vi "Lift Execute.vi"() -> ()   [LabVIEW 2017]
uses:
  Lift Control Type.ctl
  Brake Enum States.ctl
  <vilib>/Rock Robotics/WPI/DriverStation/WPI_DriverStationRobotMode2.ctl
  <vilib>/Rock Robotics/WPI/Solenoid/WPI_SolenoidValue.ctl
  Lift Notifier.ctl
  Lift Enum States.ctl
  <vilib>/Rock Robotics/WPI/ThirdParty/Phoenix-LabVIEW/Motor Controller/Controls/CTRE_Phoenix_MotorControl_ControlMode.ctl
  Lift Globals.vi
  Utility VIs/Refnum Names.vi
  Robot Global Data.vi
  <vilib>/Rock Robotics/WPI/ThirdParty/Phoenix-LabVIEW/Motor Controller/Get/CTRE_Phoenix_MotorController_GetOutputCurrent_Enhanced.vi
  <vilib>/Rock Robotics/Network Tables/NT Write Number.vi
  <vilib>/Rock Robotics/Network Tables/NT Write Boolean.vi
  <vilib>/Rock Robotics/WPI/Solenoid/WPI_SolenoidSetEnum.vi
panel:
  in  "Switch Add":dbl=1000.0 format="%#_13g"
  in  "Portal":dbl=4750.0
  out "Counts Met":bool=TRUE
  in  "Counts":i32=15
  out "Output":dbl(graph)
  in  "Graphs":bool=TRUE
  out "Position":i32(graph)
  out "Current":T1(graph)
  in  "Lift Allowable Error Down":dbl=100.0
  out "Current Error":dbl
  in  "kP Max Down":dbl=-1.0
  in  "kP Max Up":dbl=1.0
  in  "Lift Allowable Error Up":dbl=100.0
  in  "kP Down":dbl=4.18e-05
  in  "kP Up":dbl=0.00017
  out "error out 5":errorcluster
  out "error out 4":errorcluster={"status"=TRUE, "code"=-44047, "source"="Solenoid 5<LOCATION>Lift Execute.vi<CALLSTACK>Lift Execute.vi< <Periodic Tasks.vi< <Robot Main.vi"}
  out "error out 3":errorcluster={"status"=TRUE, "code"=1, "source"="Wait on Notification in Lift Execute.vi->Periodic Tasks.vi->Robot Main.vi"}
  out "error out 2":errorcluster
  out "error out":errorcluster={"status"=TRUE, "code"=1, "source"="Wait on Notification in Lift Execute.vi->Periodic Tasks.vi->Robot Main.vi"}
  in  "Deadband 2":i32=6000
  in  "Deadband 1":i32=300
  in  "Drive Up Time (ms)":u32=100
  in  "Brake Disengage Time":u32=100
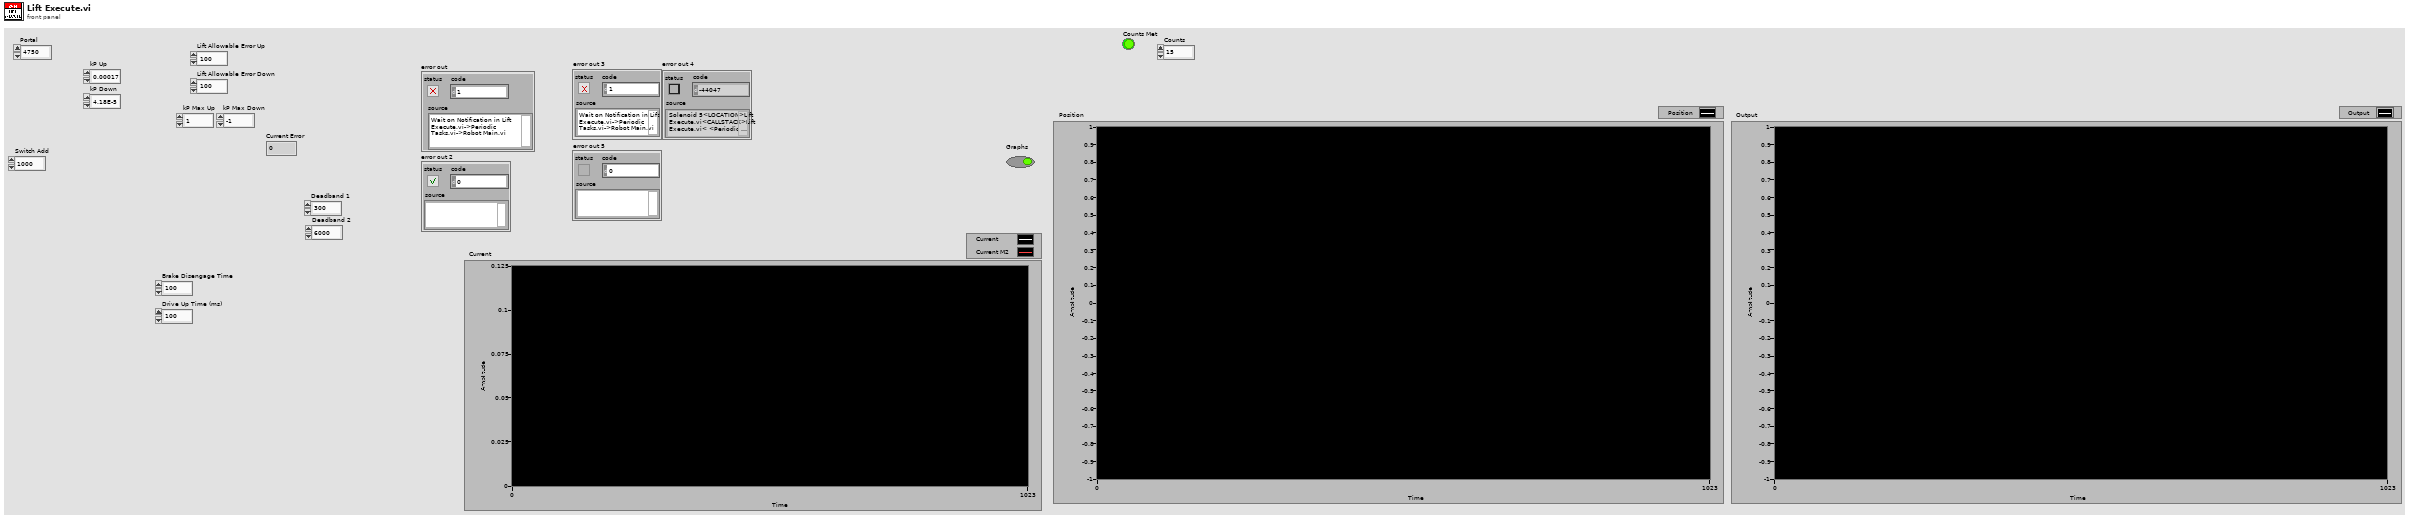
[diagram p1: front panel]
types:
  T1 = cluster{"Output Current":dbl, "Output Current":dbl}
  T2 = typedef "WPI_MotorControlDeviceRef.ctl" = cluster{"DeviceStatus":errorcluster, "Type":T3, "PWM":cluster{"PWM Channel":T4, "DeadBand":T5}, "CAN":cluster{"Device Number":u8, "SetOutput VI Ref":variant, "GetOutput VI Ref":variant, "Enable VI Ref":variant, "Disable VI Ref":variant, "Data":variant}, "Invert":bool, "DIO PWM":cluster{"PWM \"Enable\" Channel":T4, "DIOChannel":T6, "PWM Rate":dbl}}
  T3 = typedef "WPI_MotorControlType.ctl" = enum16{"PWM", "CAN", "DIO PWM"}
  T4 = typedef "FPGA_DIOPWMChannel.ctl" = enum8{"PWM 0", "PWM 1", "PWM 2", "PWM 3", "PWM 4", "PWM 5", "PWM 6", "PWM 7", "PWM 8", "PWM 9", "PWM MXP 0", "PWM MXP 1", "PWM MXP 2", "PWM MXP 3", "PWM MXP 4", "PWM MXP 5", "PWM MXP 6", "PWM MXP 7", "PWM MXP 8", "PWM MXP 9", "Invalid"}
  T5 = typedef "WPI_PWMDeadband.ctl" = cluster{"Name":string, "maxPositivePwm":i32, "minPositivePwm":i32, "centerPwm":i32, "maxNegativePwm":i32, "minNegativePwm":i32, "angularRange":u16}
  T6 = typedef "FPGA_DIOChannel.ctl" = enum8{"DIO 0", "DIO 1", "DIO 2", "DIO 3", "DIO 4", "DIO 5", "DIO 6", "DIO 7", "DIO 8", "DIO 9", "DIO MXP 0", "DIO MXP 1", "DIO MXP 2", "DIO MXP 3", "DIO MXP 4", "DIO MXP 5", "DIO MXP 6", "DIO MXP 7", "DIO MXP 8", "DIO MXP 9", "DIO MXP 10", "DIO MXP 11", "DIO MXP 12", "DIO MXP 13", "DIO MXP 14", "DIO MXP 15", "SPI Port CS1", "SPI Port CS2", "SPI Port CS3", "SPI Port MISO", "SPI Port MOSI", "Invalid"}
  T7 = typedef "WPI_SolenoidDevRef.ctl" = cluster{"DevStatus":errorcluster, "Pneumatics Control Module":u8, "Forward Solenoid Channel":T8, "Reverse Solenoid Channel":T8}
  T8 = typedef "WPI_SolenoidChannel.ctl" = enum8{"Solenoid 0", "Solenoid 1", "Solenoid 2", "Solenoid 3", "Solenoid 4", "Solenoid 5", "Solenoid 6", "Solenoid 7", "Invalid"}
  T9 = typedef "WPI_SolenoidValue.ctl" = enum16{"Off", "On", "Forward", "Reverse"}
  T10 = typedef "Lift Control Type.ctl" = enum16{"No Op", "Position", "Climb Actuation", "Manual Up", "Manual Down", "PositionAuto", "Position_kP", "Position_Delay"}
  T11 = typedef "WPI_DriverStationRobotMode2.ctl" = enum16{"Autonomous Disabled", "Autonomous Enabled", "Teleop Disabled", "Teleop Enabled", "Disconnected", "Finish", "Test Disabled", "Test Enabled", "Emergency Stopped"}
  T12 = typedef "Brake Enum States.ctl" = enum16{"Brake", "Disengage Brake", "Drive Up", "Pass Through"}
  T13 = typedef "Lift Notifier.ctl" = cluster{"Lift Control Type":T10, "Step":i32, "Set Position":T14, "Climb":bool, "Switch":bool, "Scale Low":bool, "Scale Mid":bool, "Scale High":bool, "Stow":bool, "Load":bool, "Climb Actuation":bool, "Manual Up":bool, "Manual Down":bool, "Parameter 1":dbl, "Parameter 2":dbl, "Parameter 3":dbl, "Lift Notifier":refnum<notifier>, "Exchange":bool, "Brake":bool, "Portal":bool}
  T14 = typedef "Lift Enum States.ctl" = enum16{"Climb", "Load", "Portal", "Switch", "Scale High", "Scale Mid", "Scale Low", "Exchange", "Stow", "Current Position"}
  T15 = typedef "CTRE_Phoenix_MotorControl_ControlMode.ctl" = u16
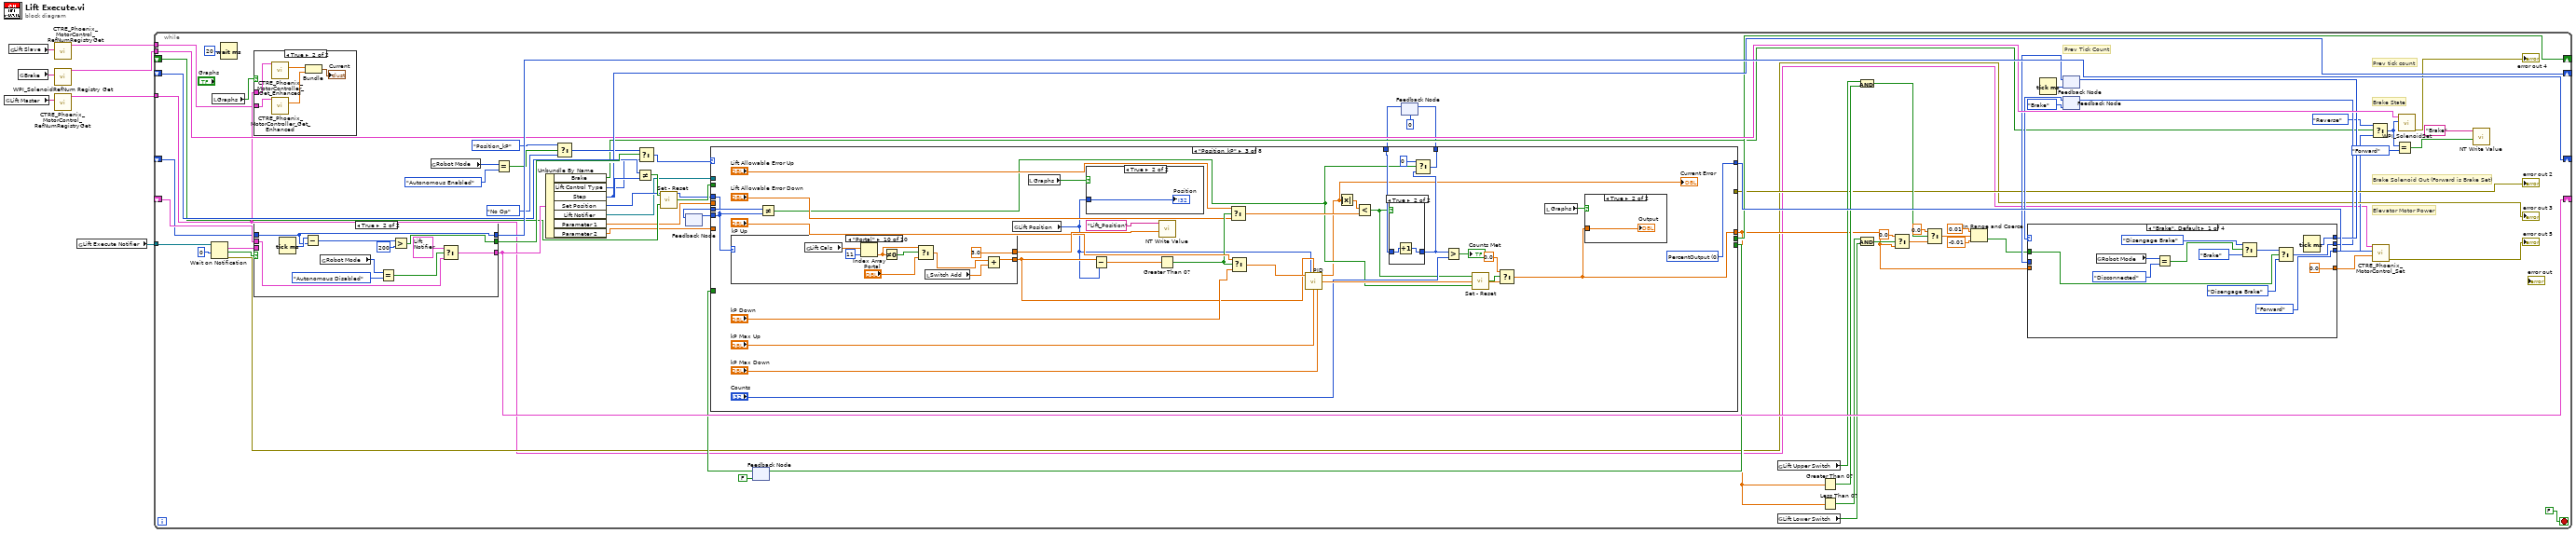
[diagram p0: block diagram]
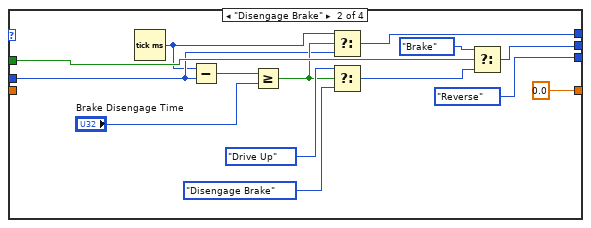
[diagram p3: hidden frame]
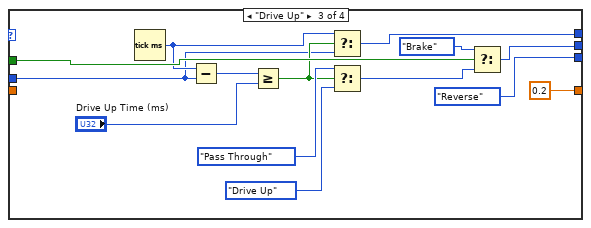
[diagram p4: hidden frame]
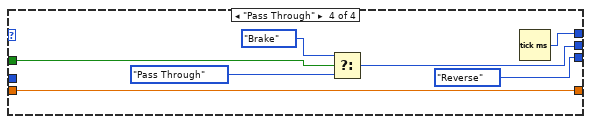
[diagram p5: hidden frame]
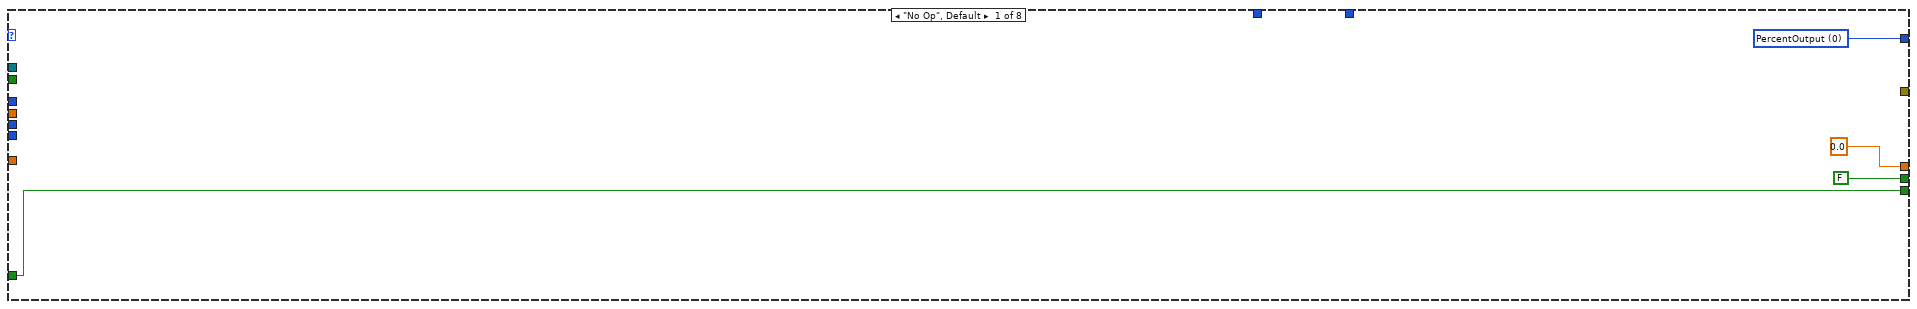
[diagram p6: hidden frame]
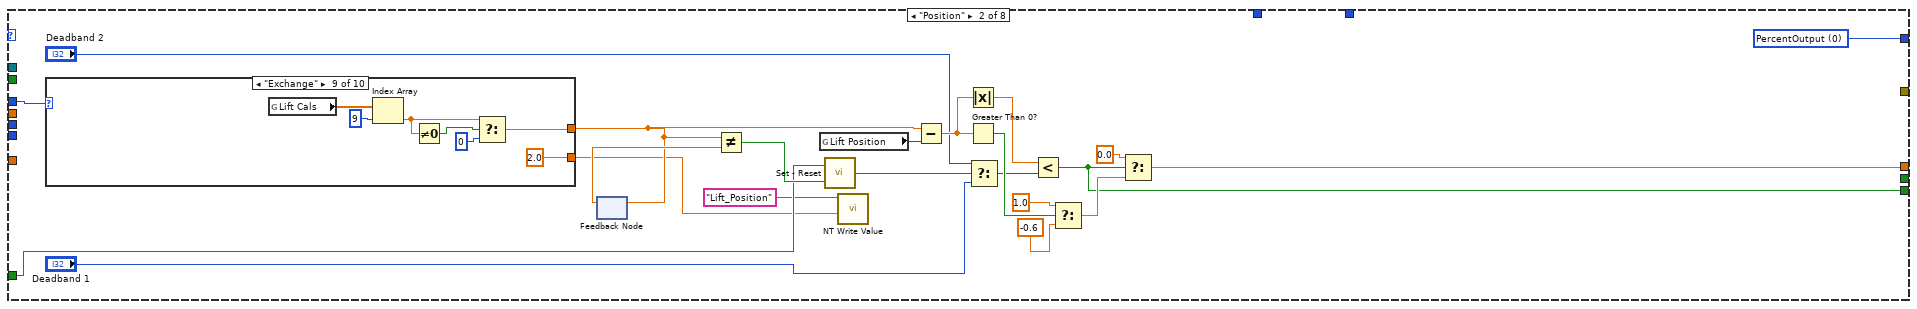
[diagram p7: hidden frame]
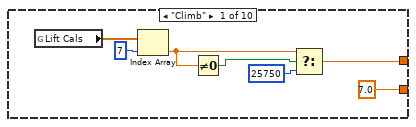
[diagram p8: hidden frame]
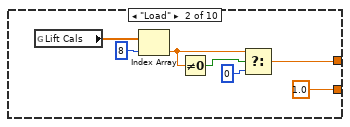
[diagram p9: hidden frame]
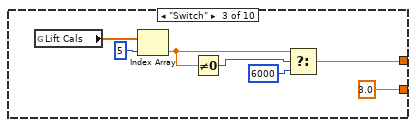
[diagram p10: hidden frame]
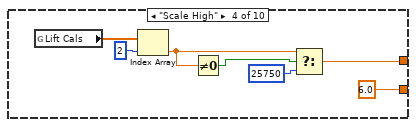
[diagram p11: hidden frame]
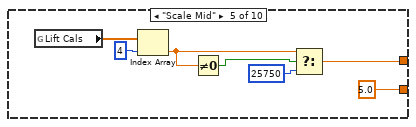
[diagram p12: hidden frame]
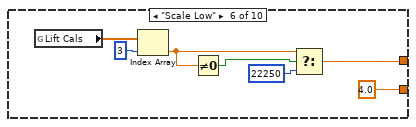
[diagram p13: hidden frame]
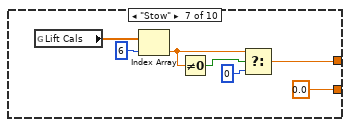
[diagram p14: hidden frame]
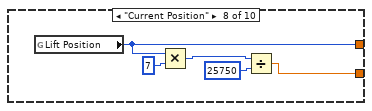
[diagram p15: hidden frame]
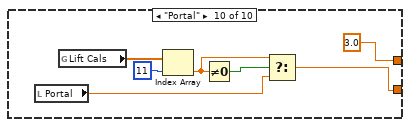
[diagram p16: hidden frame]
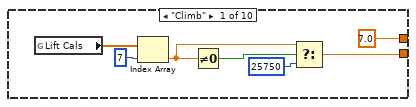
[diagram p20: hidden frame]
diagram:
  n1 = global read "Refnum Names.vi" "Lift Master"() -> (w6:string)
  n2 = global read "Refnum Names.vi" "Lift Slave"() -> (w2:string)
  n3 = global read "Refnum Names.vi" "Brake"() -> (w4:string)
  n4 = call <vilib>:"CTRE_Phoenix_MotorControl_RefNumRegistryGet.vi"("refnum name"=w2) -> ("PhoenixMotorControlDevRef"=w1:T2)  [unwired: 9 in, 1 out]
  n5 = call <vilib>:"WPI_SolenoidRefNum Registry Get.vi"("refnum name"=w4) -> ("SolenoidDevRef"=w3:T7)  [unwired: 9 in, 1 out]
  n6 = call <vilib>:"CTRE_Phoenix_MotorControl_RefNumRegistryGet.vi"("refnum name"=w6) -> ("PhoenixMotorControlDevRef"=w5:T2)  [unwired: 9 in, 1 out]
  n7 = global read "Lift Globals.vi" "Lift Execute Notifier"() -> (w7:refnum<notifier>)
  n8 = while {
    tunnel: w7 -> [w79]
    shift-right: [w68] -> _
    shift-left: _ -> [w76]
    shift-right: [w74] -> _
    shift-left: _ -> [w64]
    shift-right: [w71] -> _
    shift-left: _ -> [w72]
    tunnel: w5 -> [w15]
    tunnel: w3 -> [w65]
    shift-right: [w63] -> _
    shift-left: _ -> [w62]
    tunnel: w1 -> [w14]
    stop <- FALSE stop-if-true
    # "Elevator Motor Power"
    # "Prev tick count"
    # "Brake State"
    # "Brake Solenoid Out (Forward is Brake Set)"
    # "Prev Tick Count"
    n9 = Wait on Notification(notifier=w79, timeout in ms (-1)=0) -> (notification=w75:T13, timed out?=w77:bool, error out=→"error out 3":errorcluster)  [unwired: 2 in, 1 out]
    n10 = local read "Graphs"() -> (w13:bool)
    n11 = Wait (ms)(milliseconds to wait=u32 20) -> ()  [unwired: 1 out]
    n12 = case shown="True" w13 {
      tunnel: w15 -> [_ w86]
      tunnel: w14 -> [_ w85]
      frame False {
      }
      frame True {
        n13 = call-poly <vilib>:"CTRE_Phoenix_MotorController_Get_Enhanced.vi"("PhoenixMotorControlDevRef"=w86) -> ("Output Current"=w83:dbl)  [unwired: 12 in, 2 out]
        n14 = call-poly <vilib>:"CTRE_Phoenix_MotorController_Get_Enhanced.vi"("PhoenixMotorControlDevRef"=w85) -> ("Output Current"=w84:dbl)  [unwired: 12 in, 2 out]
        n15 = Bundle("Output Current"=w83, "Output Current"=w84) -> (→"Current":T1)  [unwired: 1 in]
      }
    }
    n16 = case shown="True" w77 {
      tunnel: w76 -> [_ w401]
      tunnel: [w391 w400] -> w68
      tunnel: w75 -> [w391 _]
      tunnel: [w390 w393] -> w74
      tunnel: w64 -> [_ w393]
      tunnel: [FALSE w396] -> w73
      frame False {
        n17 = Tick Count (ms)() -> (millisecond timer value=w390:u32)
      }
      frame True {
        n18 = Tick Count (ms)() -> (millisecond timer value=w399:u32)
        n19 = Subtract(x=w399, y=w393) -> (x-y=w398:u32)
        n20 = global read "Robot Global Data.vi" "Robot Mode"() -> (w395:T11)
        n21 = Equal?(x=w395, y=WPI_DriverStationRobotMode2."Autonomous Disabled") -> (x = y?=w402:bool)
        n22 = Greater?(x=w398, y=u32 200) -> (0:w396:bool)
        n23 = Select(t=T13 {"Lift Control Type"=enum."No Op", "Step"=0, "Set Position"=enum."Load", "Climb"=FALSE, "Switch"=FALSE, "Scale Low"=FALSE, "Scale Mid"=FALSE, "Scale High"=FALSE, "Stow"=FALSE, "Load"=FALSE, "Climb Actuation"=FALSE, "Manual Up"=FALSE, "Manual Down"=FALSE, "Parameter 1"=0.0, "Parameter 2"=0.0, "Parameter 3"=0.0, "Lift Notifier"=refnum, "Exchange"=FALSE, "Brake"=FALSE, "Portal"=FALSE} ("Lift Notifier"), s=w402, f=w401) -> (s? t:f=w400:T13)
      }
    }
    n24 = global read "Robot Global Data.vi" "Robot Mode"() -> (w33:T11)
    n25 = Equal?(x=w33, y=WPI_DriverStationRobotMode2."Autonomous Enabled") -> (x = y?=w34:bool)
    n26 = Unbundle By Name(w68) -> ("Brake"=w20:bool, "Lift Control Type"=w61:T10, "Step"=w71:i32, "Set Position"=w67:T14, "Lift Notifier"=w36:refnum<notifier>, "Parameter 1"=w28:dbl, "Parameter 2"=w16:dbl)
    n27 = Select(t=Lift_Control_Type."Position_kP", s=w34, f=Lift_Control_Type."No Op" ("t")) -> (s? t:f=w29:T10)
    n28 = Not Equal?(x=w72, y=w71) -> (x != y?=w70:bool)
    n29 = Select(t=w29, s=w73, f=w61) -> (s? t:f=w31:T10)
    n30 = call "Set - Reset.vi"("Reset"=w62, "Set"=w70) -> ("Output"=w69:bool)
    n31 = feedback #1() -> (w8:T14)  [unwired: 1 in]
    n32 = feedback #2(FALSE) -> (w49:bool)
    n33 = feedback #3(0) -> (w10:i32)
    n34 = case shown="\"Position_kP\"" w31 {
      tunnel: w69 -> [_ _ _ _ _ _ w376 w382]
      tunnel: w67 -> [_ w143 w237 _ _ _ w377 w381]
      tunnel: [0.0 ("Output") w156 w242 w338 w349 w360 w375 w385] -> w37
      tunnel: [w137 w159 w260 w344 w356 w369 w378 w388] -> w66
      tunnel: [FALSE ("notification") _ _ _ _ FALSE w374 w384] -> w63
      tunnel: [w135 w149 _ _ _ _ _ _] -> w50
      tunnel: w49 -> [w135 w145 _ _ _ _ _ _]
      tunnel: w36 -> [_ _ _ _ _ _ w372 w387]
      tunnel: w28 -> [_ _ _ _ _ _ w371 w380]
      tunnel: [_ _ _ _ _ _ w370 w386] -> w27
      tunnel: w16 -> [_ _ _ _ _ _ _ w379]
      tunnel: [_ _ w235 _ _ _ _ _] -> w11
      tunnel: w10 -> [_ _ w240 _ _ _ _ _]
      tunnel: [_ _ w237 _ _ _ _ _] -> w9
      tunnel: w8 -> [_ _ w238 _ _ _ _ _]
      frame "No Op", Default {
        w137 = T15 0 items=["PercentOutput"=0, "Position"=1, "Velocity"=2, "Current"=3, "Follower"=5, "MotionProfile"=6, "MotionMagic"=7, "MotionMagicArc"=8, "MotionProfileArc"=10, "Disabled"=15] ("Control Mode")
      }
      frame "Position" {
        w159 = T15 0 items=["PercentOutput"=0, "Position"=1, "Velocity"=2, "Current"=3, "Follower"=5, "MotionProfile"=6, "MotionMagic"=7, "MotionMagicArc"=8, "MotionProfileArc"=10, "Disabled"=15] ("Control Mode")
        n35 = case shown="\"Exchange\"" w143 {
          tunnel: [w161 w169 w175 w182 w189 w196 w205 w213 w215 3.0 ("Numeric")] -> w144
          tunnel: [7.0 1.0 3.0 6.0 5.0 4.0 0.0 w209 2.0 w223] -> w139
          frame "Climb" {
            n36 = global read "Lift Globals.vi" "Lift Cals"() -> (w166:dbl[])
            n37 = Index Array(array=w166, index=7) -> (element=w163:dbl)
            n38 = Not Equal To 0?(x=w163) -> (x != 0?=w164:bool)
            n39 = Select(t=w163, s=w164, f=25750 ("Lift Position")) -> (s? t:f=w161:dbl)
          }
          frame "Load" {
            n40 = global read "Lift Globals.vi" "Lift Cals"() -> (w173:dbl[])
            n41 = Index Array(array=w173, index=8) -> (element=w170:dbl)
            n42 = Not Equal To 0?(x=w170) -> (x != 0?=w171:bool)
            n43 = Select(t=w170, s=w171, f=0 ("Lift Position")) -> (s? t:f=w169:dbl)
          }
          frame "Switch" {
            n44 = global read "Lift Globals.vi" "Lift Cals"() -> (w180:dbl[])
            n45 = Index Array(array=w180, index=5) -> (element=w176:dbl)
            n46 = Not Equal To 0?(x=w176) -> (x != 0?=w178:bool)
            n47 = Select(t=w176, s=w178, f=6000 ("Lift Position")) -> (s? t:f=w175:dbl)
          }
          frame "Scale High" {
            n48 = global read "Lift Globals.vi" "Lift Cals"() -> (w187:dbl[])
            n49 = Index Array(array=w187, index=2) -> (element=w183:dbl)
            n50 = Not Equal To 0?(x=w183) -> (x != 0?=w185:bool)
            n51 = Select(t=w183, s=w185, f=25750 ("Lift Position")) -> (s? t:f=w182:dbl)
          }
          frame "Scale Mid" {
            n52 = global read "Lift Globals.vi" "Lift Cals"() -> (w194:dbl[])
            n53 = Index Array(array=w194, index=4) -> (element=w190:dbl)
            n54 = Not Equal To 0?(x=w190) -> (x != 0?=w192:bool)
            n55 = Select(t=w190, s=w192, f=25750 ("Lift Position")) -> (s? t:f=w189:dbl)
          }
          frame "Scale Low" {
            n56 = global read "Lift Globals.vi" "Lift Cals"() -> (w201:dbl[])
            n57 = Index Array(array=w201, index=3) -> (element=w197:dbl)
            n58 = Not Equal To 0?(x=w197) -> (x != 0?=w199:bool)
            n59 = Select(t=w197, s=w199, f=22250 ("Lift Position")) -> (s? t:f=w196:dbl)
          }
          frame "Stow" {
            n60 = global read "Lift Globals.vi" "Lift Cals"() -> (w208:dbl[])
            n61 = Index Array(array=w208, index=6) -> (element=w204:dbl)
            n62 = Not Equal To 0?(x=w204) -> (x != 0?=w206:bool)
            n63 = Select(t=w204, s=w206, f=0 ("Lift Position")) -> (s? t:f=w205:dbl)
          }
          frame "Current Position" {
            n64 = global read "Lift Globals.vi" "Lift Position"() -> (w213:i32)
            n65 = Multiply(x=w213, y=7) -> (x*y=w211:i32)
            n66 = Divide(x=w211, y=25750) -> (x/y=w209:dbl)
          }
          frame "Exchange" {
            n67 = global read "Lift Globals.vi" "Lift Cals"() -> (w220:dbl[])
            n68 = Index Array(array=w220, index=9) -> (element=w216:dbl)
            n69 = Not Equal To 0?(x=w216) -> (x != 0?=w218:bool)
            n70 = Select(t=w216, s=w218, f=0 ("Lift Position")) -> (s? t:f=w215:dbl)
          }
          frame "Portal" {
            n71 = local read "Portal"() -> (w222:dbl)
            n72 = global read "Lift Globals.vi" "Lift Cals"() -> (w227:dbl[])
            n73 = Index Array(array=w227, index=11) -> (element=w224:dbl)
            n74 = Not Equal To 0?(x=w224) -> (x != 0?=w225:bool)
            n75 = Select(t=w224, s=w225, f=w222) -> (s? t:f=w223:dbl)
          }
        }
        n76 = feedback #4() -> (w148:dbl)  [unwired: 1 in]
        n77 = feedback-in #4(w144) -> ()
        n78 = Not Equal?(x=w144, y=w148) -> (x != y?=w146:bool)
        n79 = global read "Lift Globals.vi" "Lift Position"() -> (w158:i32)
        n80 = call "Set - Reset.vi"("Reset"=w146, "Set"=w145) -> ("Output"=w147:bool)
        n81 = call-poly <vilib>:"NT Write Value.vi"("Numeric"=w139, "Name"="Lift_Position") -> ()  [unwired: 9 in, 1 out]
        n82 = Subtract(x=w144, y=w158) -> (x-y=w153:dbl)
        n83 = Absolute Value(x=w153) -> (abs(x)=w150:dbl)
        n84 = Greater Than 0?(x=w153) -> (x > 0?=w157:bool)
        n85 = Select(t="Deadband 2", s=w147, f="Deadband 1") -> (s? t:f=w151:i32)
        n86 = Less?(x=w150, y=w151) -> (x < y?=w149:bool)
        n87 = Select(t=1.0 ("f"), s=w157, f=-0.6) -> (s? t:f=w155:dbl)
        n88 = Select(t=0.0, s=w149, f=w155) -> (s? t:f=w156:dbl)
      }
      frame "Position_kP" {
        w260 = T15 0 items=["PercentOutput"=0, "Position"=1, "Velocity"=2, "Current"=3, "Follower"=5, "MotionProfile"=6, "MotionMagic"=7, "MotionMagicArc"=8, "MotionProfileArc"=10, "Disabled"=15] ("Control Mode")
        n89 = case shown="\"Portal\"" w237 {
          tunnel: [w267 w275 w281 w290 w297 w304 w313 w321 w323 w330] -> w251
          tunnel: [7.0 1.0 3.0 6.0 5.0 4.0 0.0 w317 2.0 3.0] -> w258
          frame "Climb" {
            n90 = global read "Lift Globals.vi" "Lift Cals"() -> (w272:dbl[])
            n91 = Index Array(array=w272, index=7) -> (element=w269:dbl)
            n92 = Not Equal To 0?(x=w269) -> (x != 0?=w270:bool)
            n93 = Select(t=w269, s=w270, f=25750 ("Lift Position")) -> (s? t:f=w267:dbl)
          }
          frame "Load" {
            n94 = global read "Lift Globals.vi" "Lift Cals"() -> (w279:dbl[])
            n95 = Index Array(array=w279, index=8) -> (element=w276:dbl)
            n96 = Not Equal To 0?(x=w276) -> (x != 0?=w277:bool)
            n97 = Select(t=w276, s=w277, f=0 ("Lift Position")) -> (s? t:f=w275:dbl)
          }
          frame "Switch" {
            n98 = global read "Lift Globals.vi" "Lift Cals"() -> (w288:dbl[])
            n99 = Index Array(array=w288, index=5) -> (element=w284:dbl)
            n100 = Not Equal To 0?(x=w284) -> (x != 0?=w286:bool)
            n101 = Select(t=w284, s=w286, f=6000 ("Lift Position")) -> (s? t:f=w283:dbl)
            n102 = Add(x=w283, y="Switch Add") -> (x+y=w281:dbl)
          }
          frame "Scale High" {
            n103 = global read "Lift Globals.vi" "Lift Cals"() -> (w295:dbl[])
            n104 = Index Array(array=w295, index=2) -> (element=w291:dbl)
            n105 = Not Equal To 0?(x=w291) -> (x != 0?=w293:bool)
            n106 = Select(t=w291, s=w293, f=25750 ("Lift Position")) -> (s? t:f=w290:dbl)
          }
          frame "Scale Mid" {
            n107 = global read "Lift Globals.vi" "Lift Cals"() -> (w302:dbl[])
            n108 = Index Array(array=w302, index=4) -> (element=w298:dbl)
            n109 = Not Equal To 0?(x=w298) -> (x != 0?=w300:bool)
            n110 = Select(t=w298, s=w300, f=25750 ("Lift Position")) -> (s? t:f=w297:dbl)
          }
          frame "Scale Low" {
            n111 = global read "Lift Globals.vi" "Lift Cals"() -> (w309:dbl[])
            n112 = Index Array(array=w309, index=3) -> (element=w305:dbl)
            n113 = Not Equal To 0?(x=w305) -> (x != 0?=w307:bool)
            n114 = Select(t=w305, s=w307, f=22250 ("Lift Position")) -> (s? t:f=w304:dbl)
          }
          frame "Stow" {
            n115 = global read "Lift Globals.vi" "Lift Cals"() -> (w316:dbl[])
            n116 = Index Array(array=w316, index=6) -> (element=w312:dbl)
            n117 = Not Equal To 0?(x=w312) -> (x != 0?=w314:bool)
            n118 = Select(t=w312, s=w314, f=0 ("Lift Position")) -> (s? t:f=w313:dbl)
          }
          frame "Current Position" {
            n119 = global read "Lift Globals.vi" "Lift Position"() -> (w321:i32)
            n120 = Multiply(x=w321, y=7) -> (x*y=w319:i32)
            n121 = Divide(x=w319, y=25750) -> (x/y=w317:dbl)
          }
          frame "Exchange" {
            n122 = global read "Lift Globals.vi" "Lift Cals"() -> (w328:dbl[])
            n123 = Index Array(array=w328, index=9) -> (element=w324:dbl)
            n124 = Not Equal To 0?(x=w324) -> (x != 0?=w326:bool)
            n125 = Select(t=w324, s=w326, f=0 ("Lift Position")) -> (s? t:f=w323:dbl)
          }
          frame "Portal" {
            n126 = global read "Lift Globals.vi" "Lift Cals"() -> (w336:dbl[])
            n127 = Index Array(array=w336, index=11) -> (element=w333:dbl)
            n128 = Not Equal To 0?(x=w333) -> (x != 0?=w334:bool)
            n129 = Select(t=w333, s=w334, f="Portal") -> (s? t:f=w331:dbl)
            n130 = local read "Switch Add"() -> (w329:dbl)
            n131 = Add(x=w331, y=w329) -> (x+y=w330:dbl)
          }
        }
        n132 = Not Equal?(x=w238, y=w237) -> (x != y?=w232:bool)
        n133 = global read "Lift Globals.vi" "Lift Position"() -> (w245:i32)
        n134 = local read "Graphs"() -> (w244:bool)
        n135 = case shown="True" w244 {
          tunnel: w245 -> [_ w265]
          frame False {
          }
          frame True {
            "Position" <- w265
          }
        }
        n136 = Subtract(x=w251, y=w245) -> (x-y=w252:dbl)
        n137 = Greater Than 0?(x=w252) -> (x > 0?=w248:bool)
        n138 = call-poly <vilib>:"NT Write Value.vi"("Numeric"=w258, "Name"="Lift_Position") -> ()  [unwired: 9 in, 1 out]
        n139 = Select(t="Lift Allowable Error Up", s=w248, f="Lift Allowable Error Down") -> (s? t:f=w243:dbl)
        n140 = Select(t="kP Up", s=w248, f="kP Down") -> (s? t:f=w255:dbl)
        n141 = call "PID.vi"("Kp"=w255, "Process Variable"=w245, "Goal"=w251, "Max Ouput"="kP Max Up", "Min Output"="kP Max Down") -> ("Current Error"=w229:dbl, "Command"=w256:dbl)  [unwired: 8 in, 1 out]
        "Current Error" <- w229
        n142 = Absolute Value(x=w229) -> (abs(x)=w228:dbl)
        n143 = Less?(x=w228, y=w243) -> (x < y?=w230:bool)
        n144 = case shown="True" w230 {
          tunnel: [w261 w263] -> w236
          tunnel: w240 -> [w261 w262]
          frame False {
          }
          frame True {
            n145 = Increment(x=w262) -> (x+1=w263:i32)
          }
        }
        n146 = Select(t=0, s=w232, f=w236) -> (s? t:f=w235:i32)
        n147 = Greater?(x=w236, y="Counts") -> (0:→"Counts Met":bool)
        n148 = call "Set - Reset.vi"("Reset"=w232, "Set"=w230) -> ("Output"=w233:bool)
        n149 = Select(t=0.0, s=w233, f=w256) -> (s? t:f=w242:dbl)
        n150 = local read "Graphs"() -> (w241:bool)
        n151 = case shown="True" w241 {
          tunnel: w242 -> [_ w264]
          frame False {
          }
          frame True {
            "Output" <- w264
          }
        }
      }
      frame "Climb Actuation" {
        w344 = T15 0 items=["PercentOutput"=0, "Position"=1, "Velocity"=2, "Current"=3, "Follower"=5, "MotionProfile"=6, "MotionMagic"=7, "MotionMagicArc"=8, "MotionProfileArc"=10, "Disabled"=15] ("Control Mode")
        n152 = global read "Lift Globals.vi" "Lift Cals"() -> (w343:dbl[])
        n153 = Index Array(array=w343, index=10) -> (element=w340:dbl)
        n154 = Not Equal To 0?(x=w340) -> (x != 0?=w341:bool)
        n155 = Select(t=w340, s=w341, f=-0.6) -> (s? t:f=w338:dbl)
      }
      frame "Manual Up" {
        w356 = T15 0 items=["PercentOutput"=0, "Position"=1, "Velocity"=2, "Current"=3, "Follower"=5, "MotionProfile"=6, "MotionMagic"=7, "MotionMagicArc"=8, "MotionProfileArc"=10, "Disabled"=15] ("Control Mode")
        n156 = global read "Lift Globals.vi" "Lift Cals"() -> (w354:dbl[])
        n157 = Index Array(array=w354, index=0) -> (element=w351:dbl)
        n158 = global read "Robot Global Data.vi" "Robot Mode"() -> (w347:T11)
        n159 = Not Equal To 0?(x=w351) -> (x != 0?=w353:bool)
        n160 = Equal?(x=w347, y=WPI_DriverStationRobotMode2."Test Enabled") -> (x = y?=w346:bool)
        n161 = Select(t=w351, s=w353, f=0.3) -> (s? t:f=w350:dbl)
        n162 = Select(t=w350, s=w346, f=0.4) -> (s? t:f=w349:dbl)
      }
      frame "Manual Down" {
        w369 = T15 0 items=["PercentOutput"=0, "Position"=1, "Velocity"=2, "Current"=3, "Follower"=5, "MotionProfile"=6, "MotionMagic"=7, "MotionMagicArc"=8, "MotionProfileArc"=10, "Disabled"=15] ("Control Mode")
        n163 = global read "Lift Globals.vi" "Lift Cals"() -> (w366:dbl[])
        n164 = Index Array(array=w366, index=1) -> (element=w363:dbl)
        n165 = global read "Robot Global Data.vi" "Robot Mode"() -> (w361:T11)
        n166 = Not Equal To 0?(x=w363) -> (x != 0?=w365:bool)
        n167 = Equal?(x=w361, y=WPI_DriverStationRobotMode2."Test Enabled") -> (x = y?=w358:bool)
        n168 = Select(t=w363, s=w365, f=-0.1) -> (s? t:f=w359:dbl)
        n169 = Select(t=w359, s=w358, f=-0.2) -> (s? t:f=w360:dbl)
      }
      frame "PositionAuto" {
        w378 = T15 0 items=["PercentOutput"=0, "Position"=1, "Velocity"=2, "Current"=3, "Follower"=5, "MotionProfile"=6, "MotionMagic"=7, "MotionMagicArc"=8, "MotionProfileArc"=10, "Disabled"=15] ("Control Mode")
        n170 = call "Command Lift.vi"("Startup"=w376, "Timeout"=w371, "Set Position"=w377) -> ("Lift Out"=w375:dbl, "Reinit"=w374:bool, "Completed"=w373:bool)  [unwired: 6 in]
        n171 = Send Notification(notification=w373, notifier=w372) -> (error out=w370:errorcluster)  [unwired: 1 in, 1 out]
      }
      frame "Position_Delay" {
        w388 = T15 0 items=["PercentOutput"=0, "Position"=1, "Velocity"=2, "Current"=3, "Follower"=5, "MotionProfile"=6, "MotionMagic"=7, "MotionMagicArc"=8, "MotionProfileArc"=10, "Disabled"=15] ("Control Mode")
        n172 = call "Command Lift Delay.vi"("Startup"=w382, "Distance"=w379, "Timeout"=w380, "Set Position"=w381) -> ("Lift Out"=w385:dbl, "Reinit"=w384:bool, "Completed"=w383:bool)  [unwired: 5 in]
        n173 = Send Notification(notification=w383, notifier=w387) -> (error out=w386:errorcluster)  [unwired: 1 in, 1 out]
      }
    }
    "error out 2" <- w27
    n174 = feedback-in #1(w9) -> ()
    n175 = feedback-in #2(w50) -> ()
    n176 = feedback-in #3(w11) -> ()
    n177 = global read "Lift Globals.vi" "Lift Upper Switch"() -> (w46:bool)
    n178 = global read "Lift Globals.vi" "Lift Lower Switch"() -> (w40:bool)
    n179 = Greater Than 0?(x=w37) -> (x > 0?=w47:bool)
    n180 = Less Than 0?(x=w37) -> (x < 0?=w41:bool)
    n181 = And(x=w46, y=w47) -> (x .and. y?=w45:bool)
    n182 = And(x=w41, y=w40) -> (x .and. y?=w39:bool)
    n183 = Select(t=0.0, s=w39, f=w37) -> (s? t:f=w42:dbl)
    n184 = Select(t=0.0, s=w45, f=w42) -> (s? t:f=w44:dbl)
    n185 = In Range and Coerce(upper limit=0.01, x=w44, lower limit=-0.01) -> (In Range?=w53:bool)  [unwired: 1 out]
    n186 = Tick Count (ms)() -> (millisecond timer value=w57:u32)
    n187 = feedback #5(w57) -> (w56:u32)
    n188 = feedback #6(Brake_Enum_States."Brake") -> (w59:T12)
    n189 = case shown="\"Brake\", Default" w59 {
      tunnel: [w97 w105 w124 w129] -> w52
      tunnel: [w96 w101 w115 w128] -> w58
      tunnel: w56 -> [_ w103 w116 _]
      tunnel: w53 -> [w95 w106 w126 w132]
      tunnel: [WPI_SolenoidValue."Forward" ("Value") WPI_SolenoidValue."Reverse" ("Value") WPI_SolenoidValue."Reverse" ("Value") WPI_SolenoidValue."Reverse" ("Value")] -> w22
      tunnel: [0.0 ("f") 0.0 ("f") 0.2 w133] -> w51
      tunnel: w37 -> [_ _ _ w133]
      frame "Brake", Default {
        n190 = global read "Robot Global Data.vi" "Robot Mode"() -> (w90:T11)
        n191 = Equal?(x=w90, y=WPI_DriverStationRobotMode2."Disconnected") -> (x = y?=w88:bool)
        n192 = Select(t=Brake_Enum_States."Disengage Brake", s=w88, f=Brake_Enum_States."Brake") -> (s? t:f=w91:T12)
        n193 = Select(t=w91, s=w95, f=Brake_Enum_States."Disengage Brake") -> (s? t:f=w97:T12)
        n194 = Tick Count (ms)() -> (millisecond timer value=w96:u32)
      }
      frame "Disengage Brake" {
        n195 = Tick Count (ms)() -> (millisecond timer value=w102:u32)
        n196 = Subtract(x=w102, y=w103) -> (x-y=w112:u32)
        n197 = Greater Or Equal?(x=w112, y="Brake Disengage Time") -> (x >= y?=w104:bool)
        n198 = Select(t=w102, s=w104, f=w103) -> (s? t:f=w101:u32)
        n199 = Select(t=Brake_Enum_States."Drive Up", s=w104, f=Brake_Enum_States."Disengage Brake") -> (s? t:f=w107:T12)
        n200 = Select(t=Brake_Enum_States."Brake", s=w106, f=w107) -> (s? t:f=w105:T12)
      }
      frame "Drive Up" {
        n201 = Tick Count (ms)() -> (millisecond timer value=w117:u32)
        n202 = Subtract(x=w117, y=w116) -> (x-y=w123:u32)
        n203 = Greater Or Equal?(x=w123, y="Drive Up Time (ms)") -> (x >= y?=w118:bool)
        n204 = Select(t=w117, s=w118, f=w116) -> (s? t:f=w115:u32)
        n205 = Select(t=Brake_Enum_States."Pass Through", s=w118, f=Brake_Enum_States."Drive Up") -> (s? t:f=w119:T12)
        n206 = Select(t=Brake_Enum_States."Brake", s=w126, f=w119) -> (s? t:f=w124:T12)
      }
      frame "Pass Through" {
        n207 = Select(t=Brake_Enum_States."Brake", s=w132, f=Brake_Enum_States."Pass Through") -> (s? t:f=w129:T12)
        n208 = Tick Count (ms)() -> (millisecond timer value=w128:u32)
      }
    }
    n209 = feedback-in #5(w58) -> ()
    n210 = feedback-in #6(w52) -> ()
    n211 = Select(t=WPI_SolenoidValue."Reverse", s=w20, f=w22) -> (s? t:f=w19:T9)
    n212 = call <vilib>:"CTRE_Phoenix_MotorControl_Set.vi"("Output"=w51, "Control Mode"=w66, "PhoenixMotorControlDevRef"=w15) -> ("error out"=→"error out 5":errorcluster)  [unwired: 7 in, 1 out]
    n213 = Equal?(x=w19, y=WPI_SolenoidValue."Forward") -> (x = y?=w26:bool)
    n214 = call-poly <vilib>:"WPI_SolenoidSet.vi"("Value"=w19, "SolenoidDevRef"=w65) -> ("error out"=→"error out 4":errorcluster)  [unwired: 8 in, 1 out]
    n215 = call-poly <vilib>:"NT Write Value.vi"("Boolean"=w26, "Name"="Brake") -> ()  [unwired: 9 in, 1 out]
  }
